vi "Dispense.vi"() -> ()   [LabVIEW 2016]
uses:
  Classes/Controller/Dispenser/Ultimus V/Ultimus V.lvclass
panel:
  in  "Pressure":i16=30
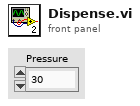
[diagram p1: front panel]
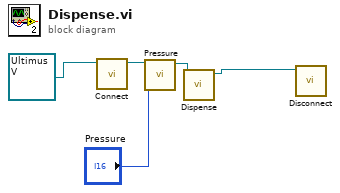
[diagram p0: block diagram]
diagram:
  n1 = call-dynamic "Connect.vi"("Ultimus V in"=refnum<class "Ultimus V.lvclass"> refnum ("Ultimus V.lvclass")) -> ("Ultimus V out"=w3:refnum<class "Ultimus V.lvclass">)  [unwired: 9 in, 1 out]
  n2 = call-dynamic "Pressure.vi"("Pressure"="Pressure", "Ultimus V in"=w3) -> ("Ultimus V out"=w2:refnum<class "Ultimus V.lvclass">)  [unwired: 8 in, 1 out]
  n3 = call-dynamic "Dispense.vi"("Ultimus V in"=w2) -> ("Ultimus V out"=w4:refnum<class "Ultimus V.lvclass">)  [unwired: 9 in, 1 out]
  n4 = call-dynamic "Disconnect.vi"("Ultimus V in"=w4) -> ()  [unwired: 9 in, 1 out]
